vi "sort1Darray.vi"(11 "Array":dbl[](array[numeric])) -> (0 "indices":dbl[](array[numeric]), 3 "sortedVals":dbl[](array[numeric]))   [LabVIEW 2010]
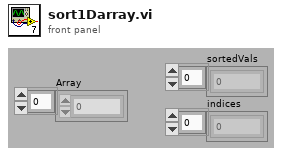
[diagram p1: front panel]
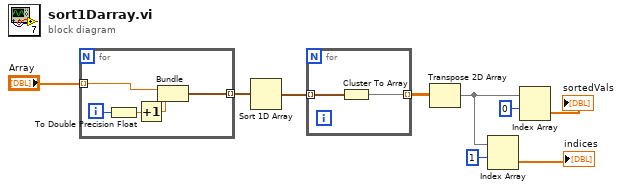
[diagram p0: block diagram]
diagram:
  n1 = for {
    tunnel: "Array" -> [w14] mode=indexing
    tunnel: [w12] -> w8 mode=indexing
    i -> [w13]
    n2 = To Double Precision Float(number=w13) -> (double precision float=w11:dbl)
    n3 = Increment(x=w11) -> (x+1=w10:dbl)
    n4 = Bundle(w14, w10) -> (w12:cluster{dbl, dbl})  [unwired: 1 in]
  }
  n5 = Sort 1D Array(array=w8) -> (sorted array=w7:cluster{dbl, dbl}[])
  n6 = for {
    tunnel: w7 -> [w16] mode=indexing
    tunnel: [w15] -> w6 mode=indexing
    n7 = Cluster To Array(cluster=w16) -> (array=w15:dbl[])
  }
  n8 = Transpose 2D Array(2D array=w6) -> (transposed array=w4:dbl[][])
  n9 = Index Array(array=w4, index (row)=1) -> (element=→"indices":dbl[])  [unwired: 1 in]
  n10 = Index Array(array=w4, index (row)=0) -> (element=→"sortedVals":dbl[])  [unwired: 1 in]
